vi "PA Get Current Data.vi"(7 "BufferSize":i32, 9 "pCurrent":dbl[](array[numeric])=array[4097 elements], 10 "Channel":i32, 11 "DevHandle":i32) -> (1 "pCurrent out":dbl[](array[numeric]), 3 "function return":i32)   [LabVIEW 2010, in "power_analyzer.lvlib"]
doc: "int WINAPI PA_GetCurrentData(int DevHandle,int Channel,double *pCurrent,int BufferSize);"
uses:
  power_analyzer.lvlib
  USB2XXX/trunk/USB2XXX/USB2XXX/vs2010/Release/USB2XXX.dll
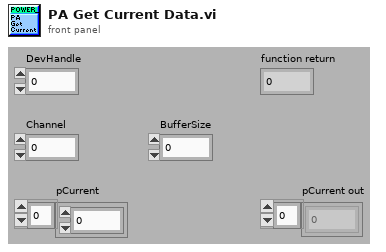
[diagram p1: front panel]
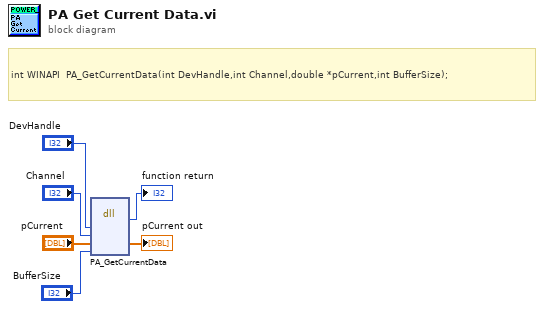
[diagram p0: block diagram]
diagram:
  # "int WINAPI  PA_GetCurrentData(int DevHandle,int Channel,double *pCurrent,int BufferSize);"
  n1 = dll-call lib="E:/Projects/USB2XXX/trunk/USB2XXX/USB2XXX/vs2010/Release/USB2XXX.*" fn="PA_GetCurrentData"("DevHandle"="DevHandle", "Channel"="Channel", "pCurrent"="pCurrent", "BufferSize"="BufferSize") -> (→"function return":i32, "pCurrent"=→"pCurrent out":dbl[])  [unwired: 6 in, 2 out]
